vi "Write Word Over 2 Addresses.vi"(7 "Address number (0)":u8, 8 "error in (no error)":errorcluster, 9 "Parameter (0)":u8, 10 "Motor ID (0)":u8, 11 "Dynamixel Motor in":refnum<class "Dynamixel Motor.lvclass">) -> (0 "error out":errorcluster, 3 "Dynamixel Motor out":refnum<class "Dynamixel Motor.lvclass">)   [LabVIEW 2016, in "Dynamixel Motor.lvclass"]
doc: "Writes a U8 to one address of the register on the motor. This is a Low-Level VI that is used by other VIs."
uses:
  <instrlib>/Dynamixel Motor/HAIOL/Dynamixel Motor.lvclass
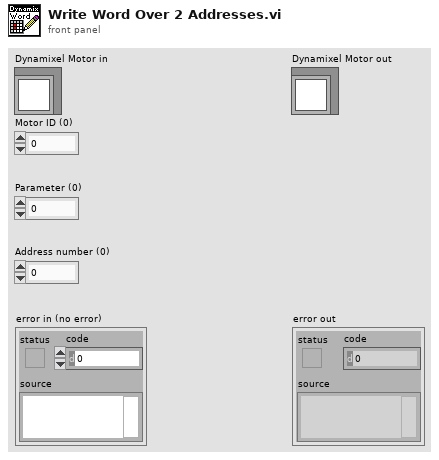
[diagram p1: front panel]
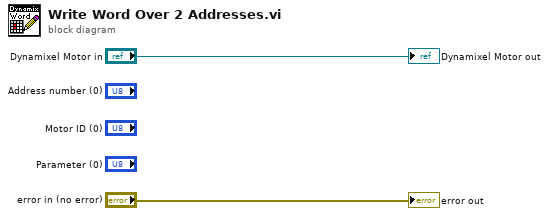
[diagram p0: block diagram]
diagram:
  "error out" <- "error in (no error)"
  "Dynamixel Motor out" <- "Dynamixel Motor in"
